vi "Coffe_Save_Files.vi"(8 "error in (no error)":errorcluster, 9 "Is Coffe Done?":bool, 10 "Coffe_Machine_ProgramData":T1) -> (0 "error out":errorcluster)   [LabVIEW 2022 SP3]
doc: "This VI create folder and file inside it (If it's already here it wont do that) and save data about what kind of coffe and when were made"
uses:
  #typedef_CM_ProgramData.ctl
  #typedef_CM_Operation.ctl
  #typedef_CM_Kind_Of_Coffe.ctl
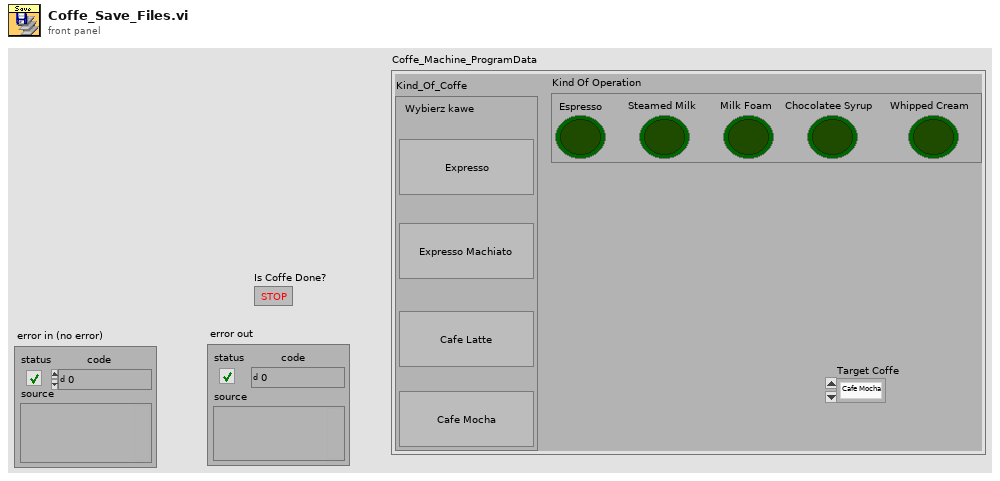
[diagram p1: front panel]
types:
  T1 = typedef "#typedef_CM_ProgramData.ctl" = cluster{"Kind Of Operation":T2, "Target Coffe":enum16{"Cafe Mocha", "Cafe Latte", "Expresso Machiato", "Expresso"}, "Kind_Of_Coffe":T3}
  T2 = typedef "#typedef_CM_Operation.ctl" = cluster{"Espresso":bool, "Steamed Milk":bool, "Milk Foam":bool, "Chocolatee Syrup":bool, "Whipped Cream":bool}
  T3 = typedef "#typedef_CM_Kind_Of_Coffe.ctl" = cluster{"Expresso":bool, "Expresso Machiato":bool, "Cafe Latte":bool, "Cafe Mocha":bool}
  T4 = enum16{"open", "replace", "create", "open or create", "replace or create", "replace or create with confirmation"}
  T5 = enum16{"Cafe Mocha", "Cafe Latte", "Expresso Machiato", "Expresso"}
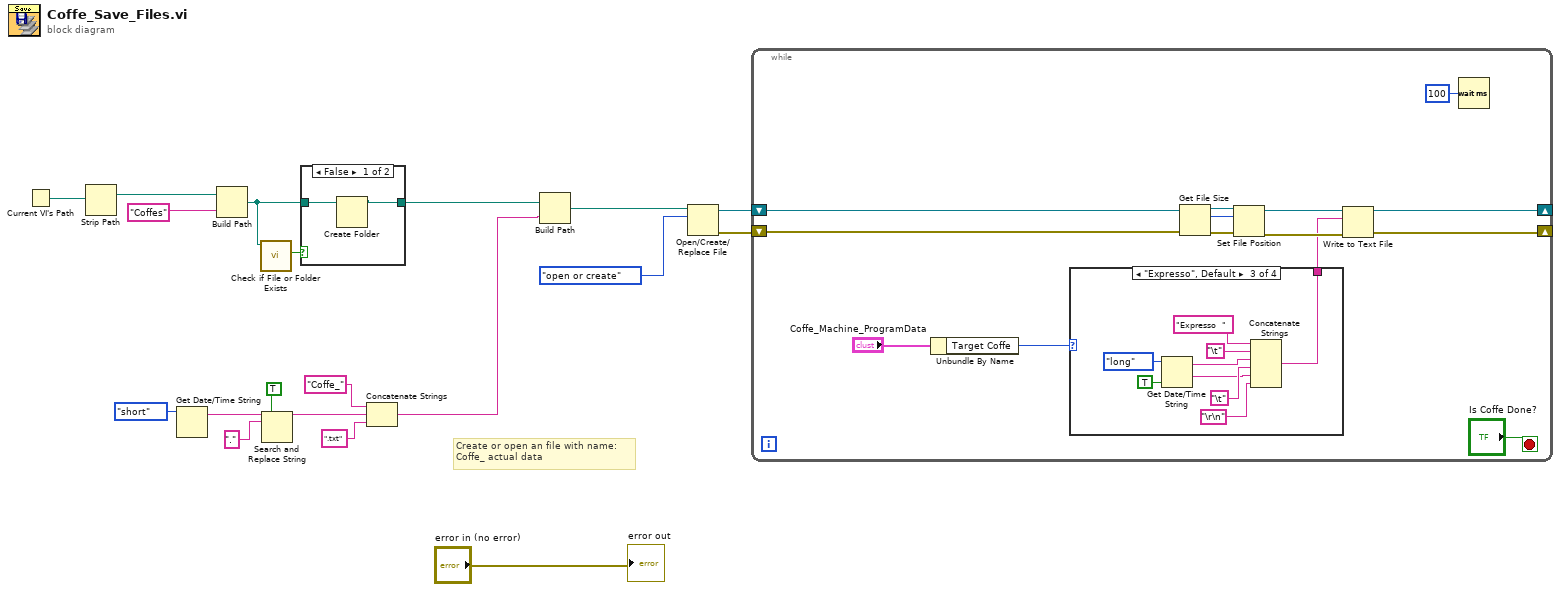
[diagram p0: block diagram]
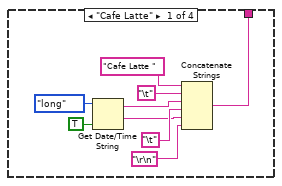
[diagram p2: hidden frame]
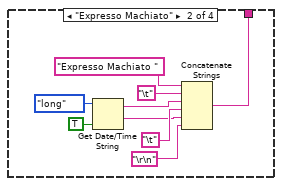
[diagram p3: hidden frame]
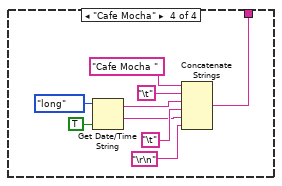
[diagram p4: hidden frame]
diagram:
  # "Create or open an file with name: \nCoffe_ actual data"
  n1 = Current VI's Path() -> (path=w19:path)
  n2 = Strip Path(path=w19) -> (stripped path=w18:path)  [unwired: 1 out]
  n3 = Get Date/Time String(date format (0)=enum16{"short", "long", "abbreviated"}."short") -> (date string=w12:string)  [unwired: 2 in, 1 out]
  n4 = Build Path(base path=w18, name or relative path="Coffes") -> (appended path=w15:path)
  n5 = call <vilib>:"Check if File or Folder Exists.vi"("path"=w15) -> ("file or folder exists?"=w16:bool)  [unwired: 8 in, 2 out]
  n6 = Search and Replace String(replace all?=TRUE ("replace all? (F)"), input string=w12, search string=".") -> (result string=w9:string)  [unwired: 5 in, 3 out]
  n7 = case shown="False" w16 {
    tunnel: w15 -> [w21 w22]
    tunnel: [w20 w22] -> w7
    frame False {
      n8 = Create Folder(path (use dialog)=w21) -> (created path=w20:path)  [unwired: 2 in, 2 out]
    }
    frame True {
    }
  }
  n9 = Concatenate Strings("Coffe_" ("string"), w9, ".txt" ("string")) -> (w6:string)
  n10 = Build Path(base path=w7, name or relative path=w6) -> (appended path=w4:path)
  n11 = Open/Create/Replace File(file path (use dialog)=w4, operation (0:open)=T4."open or create") -> (refnum out=w3:refnum<file>, error out=w2:errorcluster)  [unwired: 4 in, 1 out]
  n12 = while {
    shift-right: [w33] -> _
    shift-left: w3 -> [w35]
    shift-right: [w32] -> _
    shift-left: w2 -> [w34]
    stop <- "Is Coffe Done?" stop-if-true
    n13 = Unbundle By Name("Coffe_Machine_ProgramData") -> ("Target Coffe"=w23:T5)
    n14 = case shown="\"Expresso\", Default" w23 {
      tunnel: [w40 w49 w58 w67] -> w25
      frame "Cafe Latte" {
        n15 = Get Date/Time String(date format (0)=enum16{"short", "long", "abbreviated"}."long", want seconds? (F)=TRUE) -> (date string=w42:string, time string=w38:string)  [unwired: 1 in]
        n16 = Concatenate Strings("Cafe Latte " ("string"), "\t", w42, "\t", w38, "\r\n") -> (w40:string)
      }
      frame "Expresso Machiato" {
        n17 = Get Date/Time String(date format (0)=enum16{"short", "long", "abbreviated"}."long", want seconds? (F)=TRUE) -> (date string=w51:string, time string=w47:string)  [unwired: 1 in]
        n18 = Concatenate Strings("Expresso Machiato " ("string"), "\t", w51, "\t", w47, "\r\n") -> (w49:string)
      }
      frame "Expresso", Default {
        n19 = Get Date/Time String(date format (0)=enum16{"short", "long", "abbreviated"}."long", want seconds? (F)=TRUE) -> (date string=w60:string, time string=w56:string)  [unwired: 1 in]
        n20 = Concatenate Strings("Expresso  " ("string"), "\t", w60, "\t", w56, "\r\n") -> (w58:string)
      }
      frame "Cafe Mocha" {
        n21 = Get Date/Time String(date format (0)=enum16{"short", "long", "abbreviated"}."long", want seconds? (F)=TRUE) -> (date string=w69:string, time string=w65:string)  [unwired: 1 in]
        n22 = Concatenate Strings("Cafe Mocha " ("string"), "\t", w69, "\t", w65, "\r\n") -> (w67:string)
      }
    }
    n23 = Get File Size(file=w35, error in=w34) -> (refnum out=w30:refnum<file>, size (in bytes)=w29:i64, 0:w28:errorcluster)
    n24 = Set File Position(offset (in bytes) (0)=w29, refnum=w30, error in=w28) -> (refnum out=w27:refnum<file>, error out=w26:errorcluster)  [unwired: 1 in]
    n25 = Write to Text File(file (use dialog)=w27, text=w25, error in=w26) -> (refnum out=w33:refnum<file>, error out=w32:errorcluster)  [unwired: 1 in, 1 out]
    n26 = Wait (ms)(milliseconds to wait=u32 100) -> ()  [unwired: 1 out]
  }
  "error out" <- "error in (no error)"
